vi "The One True Carnival Main.vi"() -> ()   [LabVIEW 2013]
uses:
  <vilib>/Rock Robotics/SystemInterfaces/Typedef/FPGA_TypedefDigitalModule.ctl
  <vilib>/Rock Robotics/SystemInterfaces/DIO/FPGA_DIOChannel.ctl
  <vilib>/Rock Robotics/SystemInterfaces/DIO/FPGA_DIOPWMChannel.ctl
  motor top bottom thing.ctl
  <vilib>/Rock Robotics/WPI/MotorControl/WPI_MotorControlOpen Jaguar.vi
panel:
  out "Output":dbl
  out "s? t:f 2":dbl
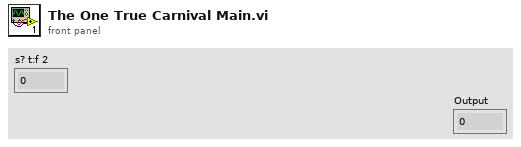
[diagram p1: front panel]
types:
  T1 = typedef "motor top bottom thing.ctl" = enum16{"Top", "Bottom Yes", "Bottom", "Upper Yes"}
  T2 = typedef "FPGA_DIOPWMChannel.ctl" = enum8{"PWM 1", "PWM 2", "PWM 3", "PWM 4", "PWM 5", "PWM 6", "PWM 7", "PWM 8", "PWM 9", "PWM 10", "Invalid"}
  T3 = typedef "FPGA_DIOChannel.ctl" = enum8{"DIO 1", "DIO 2", "DIO 3", "DIO 4", "DIO 5", "DIO 6", "DIO 7", "DIO 8", "DIO 9", "DIO 10", "DIO 11", "DIO 12", "DIO 13", "DIO 14", "Invalid"}
  T4 = typedef "FPGA_TypedefDigitalModule.ctl" = enum16{"Digital Module 1", "Digital Module 2"}
  T5 = typedef "WPI_MotorControlDeviceRef.ctl" = cluster{"DeviceStatus":errorcluster, "Type":enum16{"PWM", "CAN"}, "PWM":cluster{"Digital Module":T4, "PWM Channel":T2, "DeadBand":T6}, "CAN":cluster{"Device Number":u8, "Control Mode":T7, "Semaphore":T8, "Max Vout":dbl}, "Invert":bool, "TransformRef":T9, "InvTransformRef":T9}
  T6 = typedef "WPI_PWMDeadband.ctl" = cluster{"Name":string, "maxPositivePwm":i32, "minPositivePwm":i32, "centerPwm":i32, "maxNegativePwm":i32, "minNegativePwm":i32, "angularRange":u16}
  T7 = typedef "WPI_CANJaguar_ControlMode.ctl" = enum8{"Percent VBus", "Current", "Speed", "Position", "Voltage"}
  T8 = typedef "Semaphore RefNum" = refnum<k1>
  T9 = typedef "WPI_PWMTransform_ConPane.ctl" = refnum<vi>
  T10 = typedef "WPI_DigitalInputDevRef.ctl" = cluster{"DevStatus":errorcluster, "DIO Channel":T3, "Digital Module":T4}
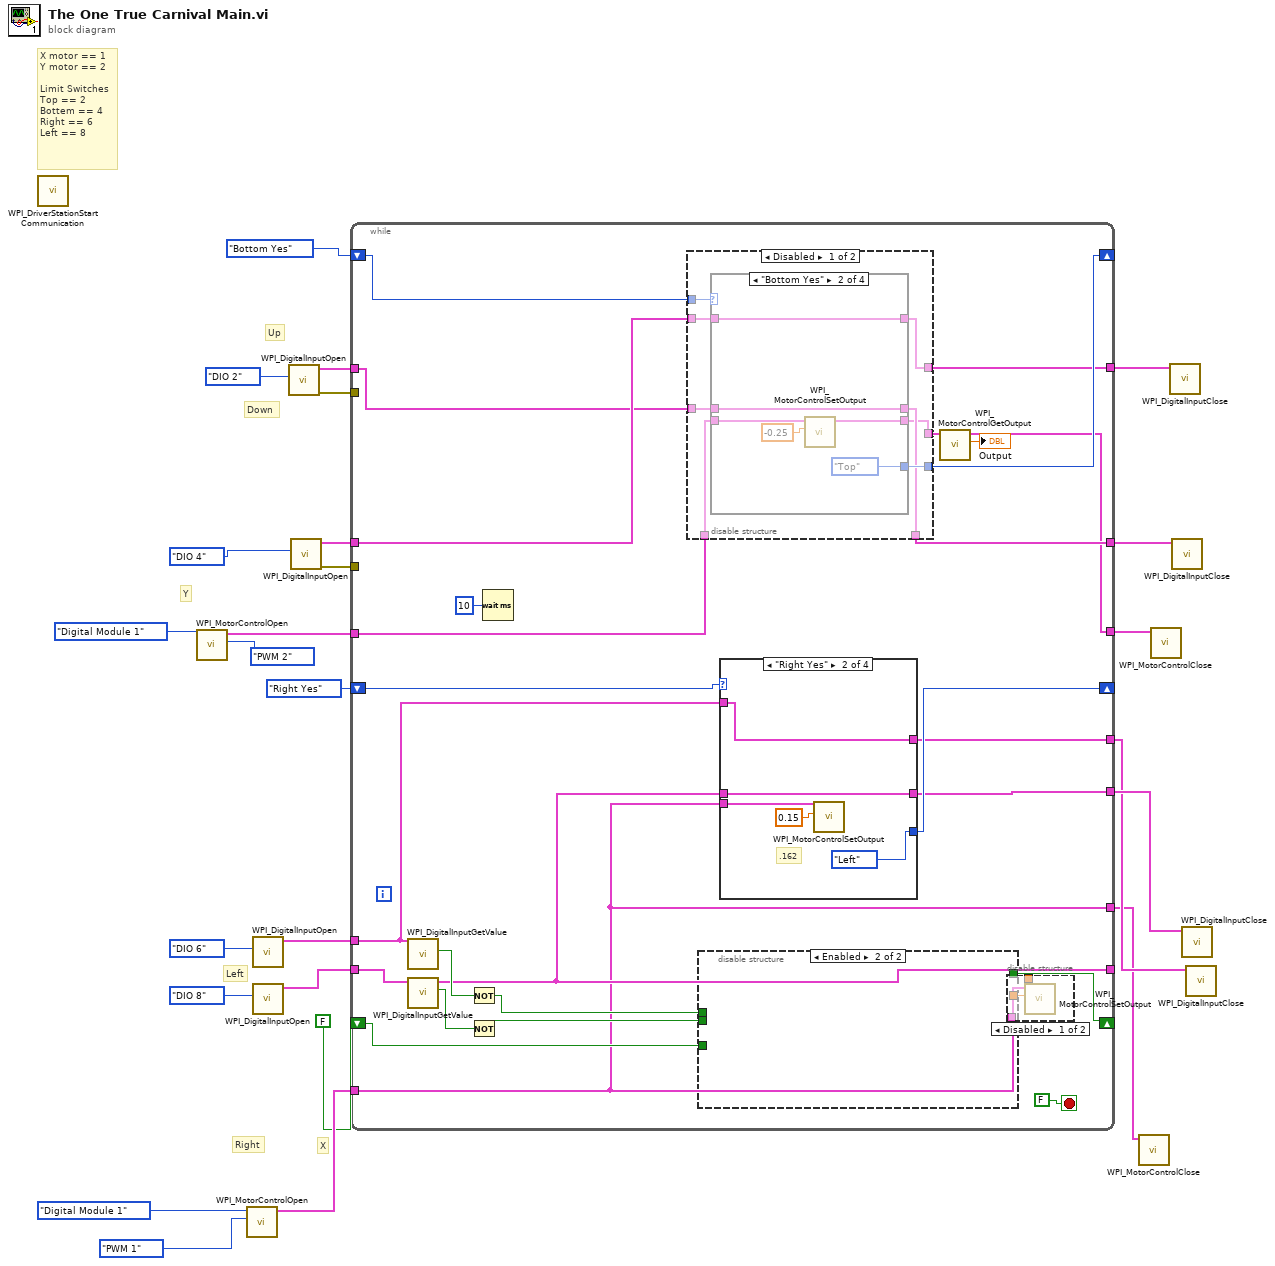
[diagram p0: block diagram]
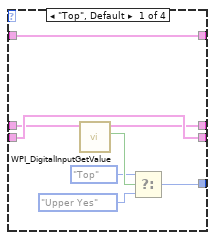
[diagram p2: hidden frame]
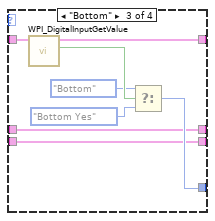
[diagram p3: hidden frame]
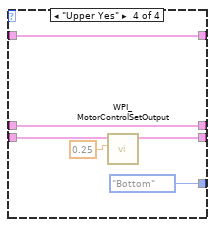
[diagram p4: hidden frame]
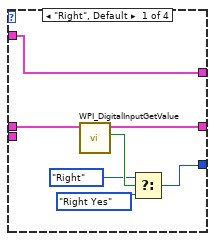
[diagram p6: hidden frame]
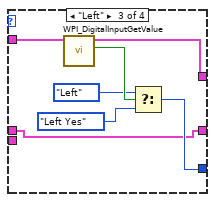
[diagram p7: hidden frame]
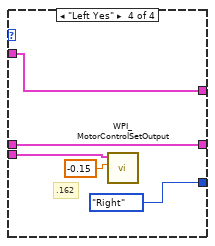
[diagram p8: hidden frame]
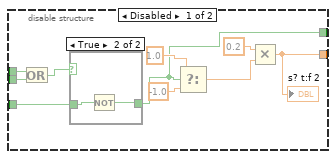
[diagram p10: hidden frame]
diagram:
  # "X"
  # "Y"
  # "Right"
  # "Left"
  # "Down"
  # "Up"
  # "X motor == 1\nY motor == 2\n\nLimit Switches\nTop == 2\nBottem == 4\nRight == 6\nLeft == 8"
  n1 = call <vilib>:"WPI_DriverStationStart Communication.vi"() -> ()  [unwired: 12 in]
  n2 = call-poly <vilib>:"WPI_MotorControlOpen.vi"("PWM Channel"=FPGA_DIOPWMChannel."PWM 2", "Digital Module (Module 1)"=FPGA_TypedefDigitalModule."Digital Module 1") -> ("MotorControlDeviceRef"=w10:T5)  [unwired: 8 in, 1 out]
  n3 = call-poly <vilib>:"WPI_MotorControlOpen.vi"("PWM Channel"=FPGA_DIOPWMChannel."PWM 1", "Digital Module (Module 1)"=FPGA_TypedefDigitalModule."Digital Module 1") -> ("MotorControlDeviceRef"=w9:T5)  [unwired: 8 in, 1 out]
  n4 = call <vilib>:"WPI_DigitalInputOpen.vi"("DIO Channel"=FPGA_DIOChannel."DIO 6") -> ("DigitalInputDevRef"=w16:T10)  [unwired: 9 in, 1 out]
  n5 = call <vilib>:"WPI_DigitalInputOpen.vi"("DIO Channel"=FPGA_DIOChannel."DIO 8") -> ("DigitalInputDevRef"=w17:T10)  [unwired: 9 in, 1 out]
  n6 = call <vilib>:"WPI_DigitalInputOpen.vi"("DIO Channel"=FPGA_DIOChannel."DIO 2") -> ("error out"=w7:errorcluster, "DigitalInputDevRef"=w14:T10)  [unwired: 9 in]
  n7 = call <vilib>:"WPI_DigitalInputOpen.vi"("DIO Channel"=FPGA_DIOChannel."DIO 4") -> ("error out"=w8:errorcluster, "DigitalInputDevRef"=w15:T10)  [unwired: 9 in]
  n8 = while {
    shift-right: [w41] -> _
    shift-left: motor_top_bottom_thing."Bottom Yes" -> [w42]
    tunnel: w17 -> [w46]
    tunnel: w16 -> [w28]
    tunnel: w15 -> [w39]
    tunnel: w14 -> [w37]
    tunnel: [w30] -> _
    tunnel: [w36] -> w13
    tunnel: [w38] -> w12
    tunnel: [w34] -> w11
    tunnel: w10 -> [w40]
    tunnel: w9 -> [w26]
    tunnel: w8 -> [_]
    tunnel: w7 -> [_]
    shift-right: [w43] -> _
    shift-left: FALSE -> [w44]
    shift-right: [w32] -> _
    shift-left: enum16{"Right", "Right Yes", "Left", "Left Yes"}."Right Yes" -> [w31]
    tunnel: [w29] -> w4
    tunnel: [w27] -> w3
    tunnel: [w26] -> w2
    stop <- FALSE stop-if-true
    n9 = call <vilib>:"WPI_DigitalInputGetValue.vi"("DigitalInputDevRef"=w28) -> ("Value"=w51:bool)  [unwired: 8 in, 2 out]
    n10 = call <vilib>:"WPI_DigitalInputGetValue.vi"("DigitalInputDevRef"=w46) -> ("Value"=w49:bool, "DigitalInputDevRef"=w30:T10)  [unwired: 8 in, 1 out]
    n11 = Not(x=w51) -> (.not. x?=w50:bool)
    n12 = Not(x=w49) -> (.not. x?=w48:bool)
    n13 = Wait (ms)(milliseconds to wait=u32 10) -> ()  [unwired: 1 out]
    n14 = disable-structure shown="Disabled" {
      disable-tunnel: w42 -> [w60 _]
      disable-tunnel: [w59 _] -> w41
      disable-tunnel: w40 -> [w58 _]
      disable-tunnel: w39 -> [w57 _]
      disable-tunnel: [w56 _] -> w38
      disable-tunnel: w37 -> [w55 _]
      disable-tunnel: [w54 _] -> w36
      disable-tunnel: [w53 _] -> w35
      frame Disabled {
        n15 = case shown="\"Bottom Yes\"" w60 {
          tunnel: [w65 motor_top_bottom_thing."Top" w79 motor_top_bottom_thing."Bottom"] -> w59
          tunnel: w58 -> [w64 w72 w78 w86]
          tunnel: [w64 w71 w78 w85] -> w53
          tunnel: w57 -> [w62 w70 w77 w84]
          tunnel: [w62 w70 w76 w84] -> w56
          tunnel: w55 -> [w63 w69 w75 w83]
          tunnel: [w61 w69 w75 w83] -> w54
          frame "Top", Default {
            n16 = call <vilib>:"WPI_DigitalInputGetValue.vi"("DigitalInputDevRef"=w63) -> ("Value"=w68:bool, "DigitalInputDevRef"=w61:T10)  [unwired: 8 in, 1 out]
            n17 = Select(t=motor_top_bottom_thing."Top", s=w68, f=motor_top_bottom_thing."Upper Yes") -> (s? t:f=w65:T1)
          }
          frame "Bottom Yes" {
            n18 = call <vilib>:"WPI_MotorControlSetOutput.vi"("Output"=-0.25, "MotorControlDevRef"=w72) -> ("MotorControlDevRef"=w71:T5)  [unwired: 7 in, 2 out]
          }
          frame "Bottom" {
            n19 = call <vilib>:"WPI_DigitalInputGetValue.vi"("DigitalInputDevRef"=w77) -> ("Value"=w82:bool, "DigitalInputDevRef"=w76:T10)  [unwired: 8 in, 1 out]
            n20 = Select(t=motor_top_bottom_thing."Bottom", s=w82, f=motor_top_bottom_thing."Bottom Yes") -> (s? t:f=w79:T1)
          }
          frame "Upper Yes" {
            n21 = call <vilib>:"WPI_MotorControlSetOutput.vi"("Output"=0.25, "MotorControlDevRef"=w86) -> ("MotorControlDevRef"=w85:T5)  [unwired: 7 in, 2 out]
          }
        }
      }
      frame Enabled {
      }
    }
    n22 = disable-structure shown="Enabled" {
      disable-tunnel: w50 -> [w124 _]
      disable-tunnel: w48 -> [w123 _]
      disable-tunnel: [w118 _] -> w47
      disable-tunnel: w44 -> [w117 _]
      disable-tunnel: [w115 _] -> w43
      frame Disabled {
        n23 = Or(x=w124, y=w123) -> (x .or. y?=w116:bool)
        n24 = case shown="True" w116 {
          tunnel: [w125 w127] -> w115
          tunnel: w117 -> [w125 w126]
          frame False {
          }
          frame True {
            n25 = Not(x=w126) -> (.not. x?=w127:bool)
          }
        }
        n26 = Select(t=1.0, s=w115, f=-1.0) -> (s? t:f=w119:dbl)
        n27 = Multiply(x=0.2, y=w119) -> (x*y=w118:dbl)
        "s? t:f 2" <- w118
      }
      frame Enabled {
      }
    }
    n28 = case shown="\"Right Yes\"" w31 {
      tunnel: [w94 enum16{"Right", "Right Yes", "Left", "Left Yes"}."Left" w106 enum16{"Right", "Right Yes", "Left", "Left Yes"}."Right"] -> w32
      tunnel: [w93 w98 w101 w109] -> w29
      tunnel: w26 -> [_ w96 _ w111]
      tunnel: w30 -> [w92 w98 w101 w109]
      tunnel: w28 -> [w89 w97 w103 w108]
      tunnel: [w89 w97 w102 w108] -> w27
      frame "Right", Default {
        n29 = call <vilib>:"WPI_DigitalInputGetValue.vi"("DigitalInputDevRef"=w92) -> ("Value"=w95:bool, "DigitalInputDevRef"=w93:T10)  [unwired: 8 in, 1 out]
        n30 = Select(t=enum16{"Right", "Right Yes", "Left", "Left Yes"}."Right", s=w95, f=enum16{"Right", "Right Yes", "Left", "Left Yes"}."Right Yes") -> (s? t:f=w94:enum16{"Right", "Right Yes", "Left", "Left Yes"})
      }
      frame "Right Yes" {
        # ".162"
        n31 = call <vilib>:"WPI_MotorControlSetOutput.vi"("Output"=0.15, "MotorControlDevRef"=w96) -> ()  [unwired: 7 in, 3 out]
      }
      frame "Left" {
        n32 = call <vilib>:"WPI_DigitalInputGetValue.vi"("DigitalInputDevRef"=w103) -> ("Value"=w107:bool, "DigitalInputDevRef"=w102:T10)  [unwired: 8 in, 1 out]
        n33 = Select(t=enum16{"Right", "Right Yes", "Left", "Left Yes"}."Left", s=w107, f=enum16{"Right", "Right Yes", "Left", "Left Yes"}."Left Yes") -> (s? t:f=w106:enum16{"Right", "Right Yes", "Left", "Left Yes"})
      }
      frame "Left Yes" {
        # ".162"
        n34 = call <vilib>:"WPI_MotorControlSetOutput.vi"("Output"=-0.15, "MotorControlDevRef"=w111) -> ()  [unwired: 7 in, 3 out]
      }
    }
    n35 = call <vilib>:"WPI_MotorControlGetOutput.vi"("MotorControlDevRef"=w35) -> ("Output"=→"Output":dbl, "MotorControlDevRef"=w34:T5)  [unwired: 8 in, 1 out]
    n36 = disable-structure shown="Disabled" {
      disable-tunnel: w47 -> [w114 _]
      disable-tunnel: w26 -> [w113 _]
      frame Disabled {
        n37 = call <vilib>:"WPI_MotorControlSetOutput.vi"("Output"=w114, "MotorControlDevRef"=w113) -> ()  [unwired: 7 in, 3 out]
      }
      frame Enabled {
      }
    }
  }
  n38 = call <vilib>:"WPI_MotorControlClose.vi"("MotorControlDevRef"=w2) -> ()  [unwired: 10 in, 1 out]
  n39 = call <vilib>:"WPI_MotorControlClose.vi"("MotorControlDevRef"=w11) -> ()  [unwired: 10 in, 1 out]
  n40 = call <vilib>:"WPI_DigitalInputClose.vi"("DigitalInputDevRef"=w12) -> ()  [unwired: 10 in, 1 out]
  n41 = call <vilib>:"WPI_DigitalInputClose.vi"("DigitalInputDevRef"=w13) -> ()  [unwired: 10 in, 1 out]
  n42 = call <vilib>:"WPI_DigitalInputClose.vi"("DigitalInputDevRef"=w4) -> ()  [unwired: 10 in, 1 out]
  n43 = call <vilib>:"WPI_DigitalInputClose.vi"("DigitalInputDevRef"=w3) -> ()  [unwired: 10 in, 1 out]
